vi "Change Numeric Constant Type.vi"(6 "VI Path":path, 7 "Data Type":T1, 8 "error in (no error)":errorcluster, 10 "Control Name":string) -> (0 "error out":errorcluster)   [LabVIEW 2018]
uses:
  <vilib>/Utility/Data Type/Type Definitions/Data Type.ctl
  <vilib>/Utility/error.llb/Error Cluster From Error Code.vi
  <vilib>/ErrorRing/Error Ring.xnode
  <vilib>/Utility/Data Type/NI_Data Type.lvlib
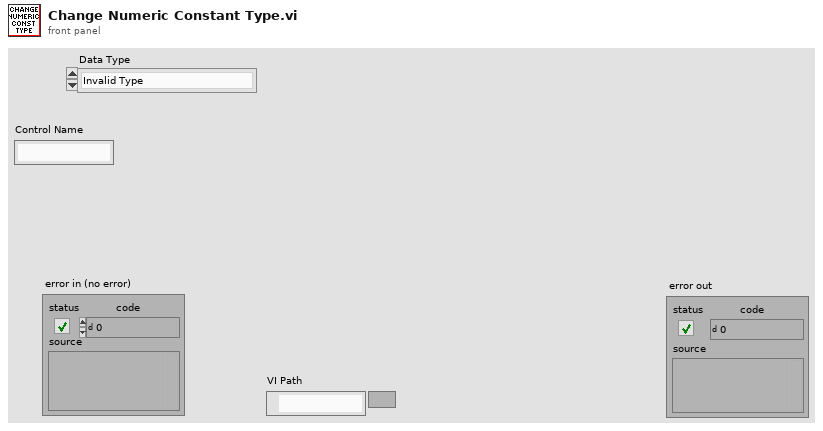
[diagram p1: front panel]
types:
  T1 = typedef "NI_Data Type.lvlib/Data Type.ctl" = enum8{"Invalid Type", "Void", "I8", "I16", "I32", "I64", "U8", "U16", "U32", "U64", "Single Float", "Double Float", "Extended Float", "Single Complex", "Double Complex", "Extended Complex", "Enum U8", "Enum U16", "Enum U32", "Enum U64", "Single Float With Unit", "Double Float With Unit", "Extended Float With Unit", "Single Complex with Unit", "Double Complex with Unit", "Extended Complex with Unit", "Boolean", "String", "Path", "Picture", "Tag", "Array", "Cluster", "Variant", "LV Variant", "Waveform", "Timestamp", "Digital Waveform", "Digital Data", "ExpressData", "Refnum", "External Data", "VI", "Poly VI", "LabVIEW Class Instance", "Fixed Point"}
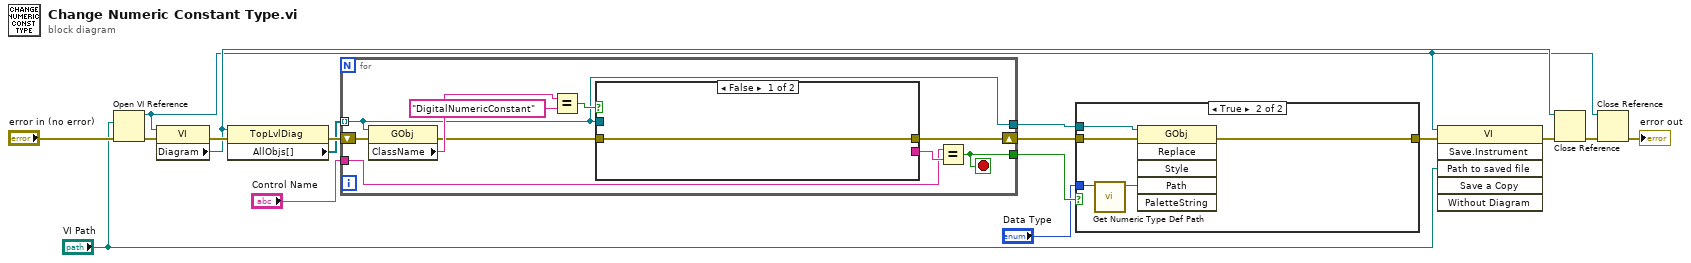
[diagram p0: block diagram]
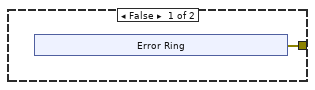
[diagram p2: hidden frame]
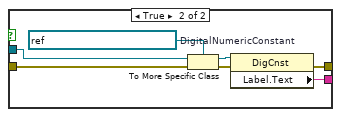
[diagram p3: hidden frame]
diagram:
  n1 = Open VI Reference(vi path="VI Path", error in (no error)="error in (no error)") -> (vi reference=w2:refnum<vi>, error out=w11:errorcluster)  [unwired: 4 in]
  n2 = property class="VI"(reference=w2, error in=w11) -> (error out=w10:errorcluster, "Diagram"=w6:refnum<vi>)  [unwired: 1 out]
  n3 = property class="TopLvlDiag"(reference=w6, error in=w10) -> (error out=w16:errorcluster, "AllObjs[]"=w7:refnum<vi>[])  [unwired: 1 out]
  n4 = for {
    tunnel: w7 -> [w18] mode=indexing
    tunnel: "Control Name" -> [w23]
    shift-right: [w20] -> w13
    shift-left: w16 -> [w21]
    tunnel: [w19] -> w15
    tunnel: [w18] -> w14
    stop <- w19 stop-if-true
    n5 = property class="GObj"(reference=w18, error in=w21) -> (error out=w22:errorcluster, "ClassName"=w27:string)  [unwired: 1 out]
    n6 = Equal?(x=w27, y="DigitalNumericConstant" ("Class Name")) -> (x = y?=w25:bool)
    n7 = case shown="False" w25 {
      tunnel: w18 -> [_ w35]
      tunnel: [_ w32] -> w24
      tunnel: w22 -> [w28 w30]
      tunnel: [w28 w29] -> w20
      frame False {
      }
      frame True {
        w34 = refnum<vi> refnum  # DigitalNumericConstant
        n8 = To More Specific Class(target class=w34, reference=w35, error in=w30) -> (specific class reference=w33:refnum<vi>, error out=w31:errorcluster)
        n9 = property class="DigCnst"(reference=w33, error in=w31) -> (error out=w29:errorcluster, "Label.Text"=w32:string)  [unwired: 1 out]
      }
    }
    n10 = Equal?(x=w23, y=w24) -> (x = y?=w19:bool)
  }
  n11 = case shown="True" w15 {
    tunnel: w14 -> [_ w46]
    tunnel: w13 -> [_ w43]
    tunnel: "Data Type" -> [_ w45]
    tunnel: [w36 w42] -> w4
    frame False {
      n12 = xnode "Error Ring"() -> ("error out"=w36:errorcluster)
    }
    frame True {
      n13 = call "Get Numeric Type Def Path.vi"("Type"=w45) -> ("Numeric Type Def Path"=w44:path)  [unwired: 10 in]
      n14 = invoke class="GObj" method="Replace"(reference=w46, error in=w43, "Path"=w44) -> (error out=w42:errorcluster)  [unwired: 3 in, 5 out]
    }
  }
  n15 = invoke class="VI" method="Save.Instrument"(reference=w2, error in=w4, "Path to saved file"="VI Path") -> (error out=w3:errorcluster)  [unwired: 3 in, 5 out]
  n16 = Close Reference(reference=w6, error in (no error)=w3) -> (error out=w8:errorcluster)
  n17 = Close Reference(reference=w2, error in (no error)=w8) -> (error out=→"error out":errorcluster)
